vi "Central_Controller_KAFB.vi"() -> ()   [LabVIEW 2019]
uses:
  <vilib>/Modbus/master/Modbus Master.lvclass
  <vilib>/Modbus/master/Create Master Instance (TCP).vi
panel:
  in  "DER List":string[](array[string])=["Capstone", "Aquion", "Tesla", "Load Bank", "Motor 1", "Simpliphi 1", "LG Chem", "Outback 1", "Outback 2", "Sunny Island", "ESS", "Fuel Cells", "Sparkplug", "Fronius", "Suny Boy", "Motor 2"]
  out "data":T1
  in  "File Name":string
  out "error out 3":errorcluster
  in  "Folder":path=path "C:/Users/administrator.STONEEDGEPOWER/Desktop/Data"
  out "ALL Status":u16[](array[numeric])
  out "ALL AC RMS Line-Neutral Voltages":sgl[][](array[numeric])
  out "SYS Current Time":dbl format="%.3f"
  out "SYS DER Index":i32
  out "ALL Frequency":sgl[](array[numeric])
  out "ALL Control Method":string[](array[string])
  out "ALL Logged":bool[](array[boolean])
  out "ALL Through Variable":sgl[](array[numeric])
  out "ALL Across Variable":sgl[](array[numeric])
  out "ALL State of Charge":sgl[](array[numeric])
  out "ALL Reactive Power":sgl[](array[numeric])
  out "ALL Real Power":sgl[](array[numeric])
  out "ALL AC RMS Line-Line Average Voltage":sgl[][](array[numeric])
  in  "Tab Control Main":enum32{"Control", "Comms Control"}(tab)
  out "DER12 Flow":i32(ring)
  out "DER12State of Charge Figure":sgl(slide) scale=0.0..100.0
  out "DER12 State of Charge":sgl format="%#.1f"
  out "DER12 Real Power":sgl format="%.1f"
  in  "DER12 Login Button":bool
  out "DER12 Logged":bool
  out "DER12 DC Voltage":sgl format="%#.1f"
  out "DER12 AC Line-Line Voltage":sgl=209.57935 format="%.1f"
  out "DER12 State":string
  in  "DER12 Control Window Button":bool
  in  "DER12 Detail Window Button":bool
  out "DER11 State of Charge":sgl format="%#.1f"
  out "DER11 Flow":i32(ring)
  in  "DER11 Detail Window Button":bool
  out "DER11 State of Charge Figure":sgl(slide) scale=0.0..100.0
  in  "DER11 Login Button":bool
  out "DER11 Across Variable":sgl format="%#.2f"
  out "DER11 logged":bool
  out "DER11 AC Line-Line Votlage":sgl format="%.1f"
  out "DER11 Real Power":sgl format="%.1f"
  out "DER11 State":string
  in  "DER11 Control Window Button":bool
  out "DER10 Flow":i32(ring)
  out "DER10 State of Charge Figure":sgl(slide) scale=0.0..100.0
  out "DER10 State of Charge":sgl format="%#.1f"
  out "DER10 Real Power":sgl format="%.1f"
  in  "DER10 Login Button":bool
  out "DER10 Logged":bool
  out "DER10 DC Voltage":sgl format="%#.1f"
  out "DER10 AC Line-Line Voltage":sgl=209.57935 format="%.1f"
  out "DER10 State":string
  in  "DER10 Control Window Button":bool
  in  "DER10 Detail Window Button":bool
  out "DER9 State of Charge":sgl format="%#.1f"
  out "DER9 Flow":i32(ring)
  in  "DER9 Detail Window Button":bool
  out "DER9 State of Charge Figure":sgl(slide) scale=0.0..100.0
  in  "DER9 Login Button":bool
  out "DER9 Across Variable":sgl format="%#.2f"
  out "DER9 logged":bool
  out "DER9 AC Line-Line Votlage":sgl format="%.1f"
  out "DER9 Real Power":sgl format="%.1f"
  out "DER9 State":string
  in  "DER9 Control Window Button":bool
  out "DER8 Flow":i32(ring)
  out "DER8 State of Charge Figure":sgl(slide) scale=0.0..100.0
  out "DER8 State of Charge":sgl format="%#.1f"
  out "DER8 Real Power":sgl format="%.1f"
  in  "DER8 Login Button":bool
  out "DER8 Logged":bool
  out "DER8 DC Voltage":sgl format="%#.1f"
  out "DER8 AC Line-Line Voltage":sgl=209.57935 format="%.1f"
  out "DER8 State":string
  in  "DER8 Control Window Button":bool
  in  "DER8 Detail Window Button":bool
  out "DER7 State of Charge":sgl format="%#.1f"
  out "DER5 State of Charge":sgl format="%#.1f"
  out "DER7 Flow":i32(ring)
  in  "DER7 Detail Window Button":bool
  out "DER7 State of Charge Figure":sgl(slide) scale=0.0..100.0
  in  "DER7 Login Button":bool
  out "DER7 Across Variable":sgl format="%#.2f"
  out "DER7 logged":bool
  out "DER7 AC Line-Line Votlage":sgl format="%.1f"
  out "DER7 Real Power":sgl format="%.1f"
  out "DER7 State":string
  in  "DER7 Control Window Button":bool
  out "DER6 Flow":i32(ring)
  out "DER6 State of Charge Figure":sgl(slide) scale=0.0..100.0
  out "DER6 State of Charge":sgl format="%#.1f"
  out "DER6 Real Power":sgl format="%.1f"
  in  "DER6 Login Button":bool
  out "DER6 Logged":bool
  out "DER6 DC Voltage":sgl format="%#.1f"
  out "DER6 AC Line-Line Voltage":sgl=209.57935 format="%.1f"
  out "DER6 State":string
  in  "DER6 Control Window Button":bool
  in  "DER6 Detail Window Button":bool
  out "DER0 State of Charge":sgl format="%.1f"
  out "DER0 State of Charge Figure":sgl(slide) scale=0.0..100.0
  out "DER5 Flow":i32(ring)
  out "DER4 Flow":i32(ring)
  out "DER3 Flow":i32(ring)
  out "DER1 Flow":i32(ring)
  out "DER0 Flow":i32(ring)
  in  "DER2 Detail Window Button":bool
  in  "DER5 Detail Window Button":bool
  out "DER4 State of Charge Figure":sgl(slide) scale=0.0..100.0
  out "DER4 State of Charge":sgl format="%#.1f"
  out "DER4 Real Power":sgl format="%.1f"
  in  "DER15 Login Button":bool
  out "DER4 Logged":bool
  out "DER4 DC Voltage":sgl format="%#.1f"
  out "DER4 AC Line-Line Voltage":sgl=209.57935 format="%.1f"
  out "DER4 State":string
  out "DER5 State of Charge Figure":sgl(slide) scale=0.0..100.0
  in  "DER0 Login Button":bool
  in  "DER2 Login Button":bool
  in  "DER1 Login Button":bool
  out "DER1 State of Charge Figure":sgl(slide) scale=0.0..100.0
  out "DER1 Real Power":sgl format="%.1f"
  out "DER1 Reactive Power":sgl format="%#.1f"
  out "DER1 AC Line-Line Voltage":sgl format="%.1f"
  out "DER0 Real Power":sgl format="%#.1f"
  out "DER0 AC Line-Line Voltage":sgl format="%#.1f"
  out "DER2 AC Line-Line Voltage":sgl format="%.1f"
  out "DER2 Real Power":sgl format="%.1f"
  out "DER0 Logged":bool
  out "DER1 Logged":bool
  out "DER2 Logged":bool
  out "DER1 State of Charge":sgl format="%.1f"
  in  "DER3 Login Button":bool
  out "DER3 Logged":bool
  out "DER3 Real Power":sgl format="%#.1f"
  out "DER3 AC Line-Line Votlage":sgl format="%#.1f"
  in  "DER5 Login Button":bool
  out "DER5 Across Variable":sgl format="%#.2f"
  out "DER5 logged":bool
  out "DER5 AC Line-Line Votlage":sgl format="%.1f"
  out "DER5 Real Power":sgl format="%.1f"
  out "DER0 State":string
  out "DER1 State":string
  out "DER2 State":string
  out "DER3 State":string
  out "DER5 State":string
  in  "DER0 Control Window Button":bool
  in  "DER0 Detail Window Button":bool
  in  "DER1 Detail Window Button":bool
  in  "DER1 Control Window Button":bool
  in  "DER2 Control Window Button":bool
  in  "DER3 Control Window Button":bool
  in  "DER5 Control Window Button":bool
  in  "DER4 Control Window Button":bool
  in  "DER3 Detail Window Button":bool
  in  "DER4 Detail Window Button":bool
  out "DER2 Control Mode":string="Slave Mode Droops"
  out "DER1 Control Mode":string="Slave Mode Droops"
  out "DER2 Flow":i32(ring)
  out "DER0 Control Mode":string="Slave Mode Droops"
  in  "Tab Control Communications":enum32{"Page 1"}(tab)
  out "ALL Error Indicator":bool[](array[boolean])
  out "ALL DER Current Error":errorcluster[](array[cluster])
  out "ALL DER Final Error":errorcluster[](array[cluster])
  in  "IP Address List":string[](array[string])=["10.1.32.65", "10.1.32.32", "10.0.1.180", "10.0.1.202", "10.0.1.189", "10.0.1.188", "10.0.1.190", "10.0.1.187", "10.0.1.195", "10.0.1.191", "10.0.1.185", "10.0.1.181", "10.0.1.201", "10.0.1.192", "10.0.1.207", "10.0.1.196"]
  in  "DER Label Name":string[](array[string])=["DER0", "DER1", "DER2", "DER3", "DER4", "DER5", "DER6", "DER7", "DER8", "DER9", "DER10", "DER11", "DER12", "DER13", "DER14", "DER15"]
  out "SYS Iteration":i32
  in  "stop":bool
  out "SYS Status":string="Reading"
  out "SYS Case":i32
  in  "Read Array":bool[](array[boolean])
  # "DER0: Heila XX, Sinamics, 10.0.8.XX\nDER1: Heila XX, Socomec, 10.0.8.XX\nDER2: Heila XX, Alencon, 10.0.8.XX\nDER3: Heila XX, Polar Power, 10.0.8.XX\nDER4: Heila XX, Nanogrid 1 \nDER5: Heila XX, Nanogrid 2\nDER6: Heila XX, Nanogrid 3\nDER7: Heila XX, Nanogrid 4 \nDER8: Heila XX, Nanogrid 5\nDER9: Heila XX, Nanogrid 6\nDER10: Heila XX, Nanogrid 7 \nDER11: Heila XX, Nanogrid 8\nDER12: Heila XX, Nanogrid 9"
  # "Nanogrid"
  # "Generators"
  # "Battery"
  # "Nanogrid"
  # "Nanogrid"
  # "Nanogrid"
  # "Nanogrid"
  # "Schaefer"
  # "EPIC + Polar Power"
  # "Sinamics + Energport"
  # "Schaefer"
  # "Schaefer"
  # "Schaefer"
  # "Schaefer"
  # "Status:"
  # "Status:"
  # "Status:"
  # "Status:"
  # "Status:"
  # "Status:"
  # "Status:"
  # "Mode:"
  # "V"
  # "V"
  # "V"
  # "V"
  # "V"
  # "KAFB Microgrid in Real Time"
  # "SoC"
  # "%"
  # "SoC"
  # "%"
  # "SoC"
  # "%"
  # "SoC"
  # "%"
  # "SoC"
  # "%"
  # "SoC"
  # "%"
  # "kW"
  # "kW"
  # "kW"
  # "kW"
  # "kW"
  # "kW"
  # "kW"
  # "Inverter"
  # "Utility Grid"
  # "kW"
  # "V"
  # "V"
  # "V"
  # "V"
  # "V"
  # "V"
  # "V"
  # "Socomec"
  # "kVAr"
  # "V"
  # "Status:"
  # "Mode:"
  # "V ="
  # "V"
  # "f ="
  # "Hz"
  # "P ="
  # "W"
  # "Q ="
  # "VAr"
  # "kW"
  # "kW"
  # "kW"
  # "kW"
  # "kW"
  # "SoC"
  # "%"
  # "V"
  # "V"
  # "V"
  # "V"
  # "V"
  # "Nanogrid"
  # "Nanogrid"
  # "Nanogrid"
  # "Nanogrid"
  # "Solar"
  # "Sinexcel"
  # "Sinexcel"
  # "Sinexcel"
  # "Sinexcel"
  # "PV + Alencon"
  # "Status:"
  # "Status:"
  # "Status:"
  # "Status:"
  # "Status:"
  # "Mode:"
  # "V"
  # "V"
  # "V"
  # "V"
  # "SoC"
  # "%"
  # "SoC"
  # "%"
  # "SoC"
  # "%"
  # "SoC"
  # "%"
  # "Program"
  # "Controllable DERs"
  # "DER0: Heila XX, Sinamics, 10.1.32.65\nDER1: Heila XX, Socomec, 10.1.32.32\nDER2: Heila XX, Alencon, 10.1.32.XX\nDER3: Heila XX, Polar Power, 10.1.32.XX\nDER4: Heila XX, Nanogrid 1, 10.1.32.45 \nDER5: Heila XX, Nanogrid 2, 10.1.32.67\nDER6: Heila XX, Nanogrid 3, 10.1.32.70\nDER7: Heila XX, Nanogrid 4, 10.1.32.100\nDER8: Heila XX, Nanogrid 5, 10.1.32.68\nDER9: Heila XX, Nanogrid 6, 10.1.32.38\nDER10: Heila XX, Nanogrid 7, 10.1.32.43\nDER11: Heila XX, Nanogrid 8\nDER12: Heila XX, Nanogrid 9"
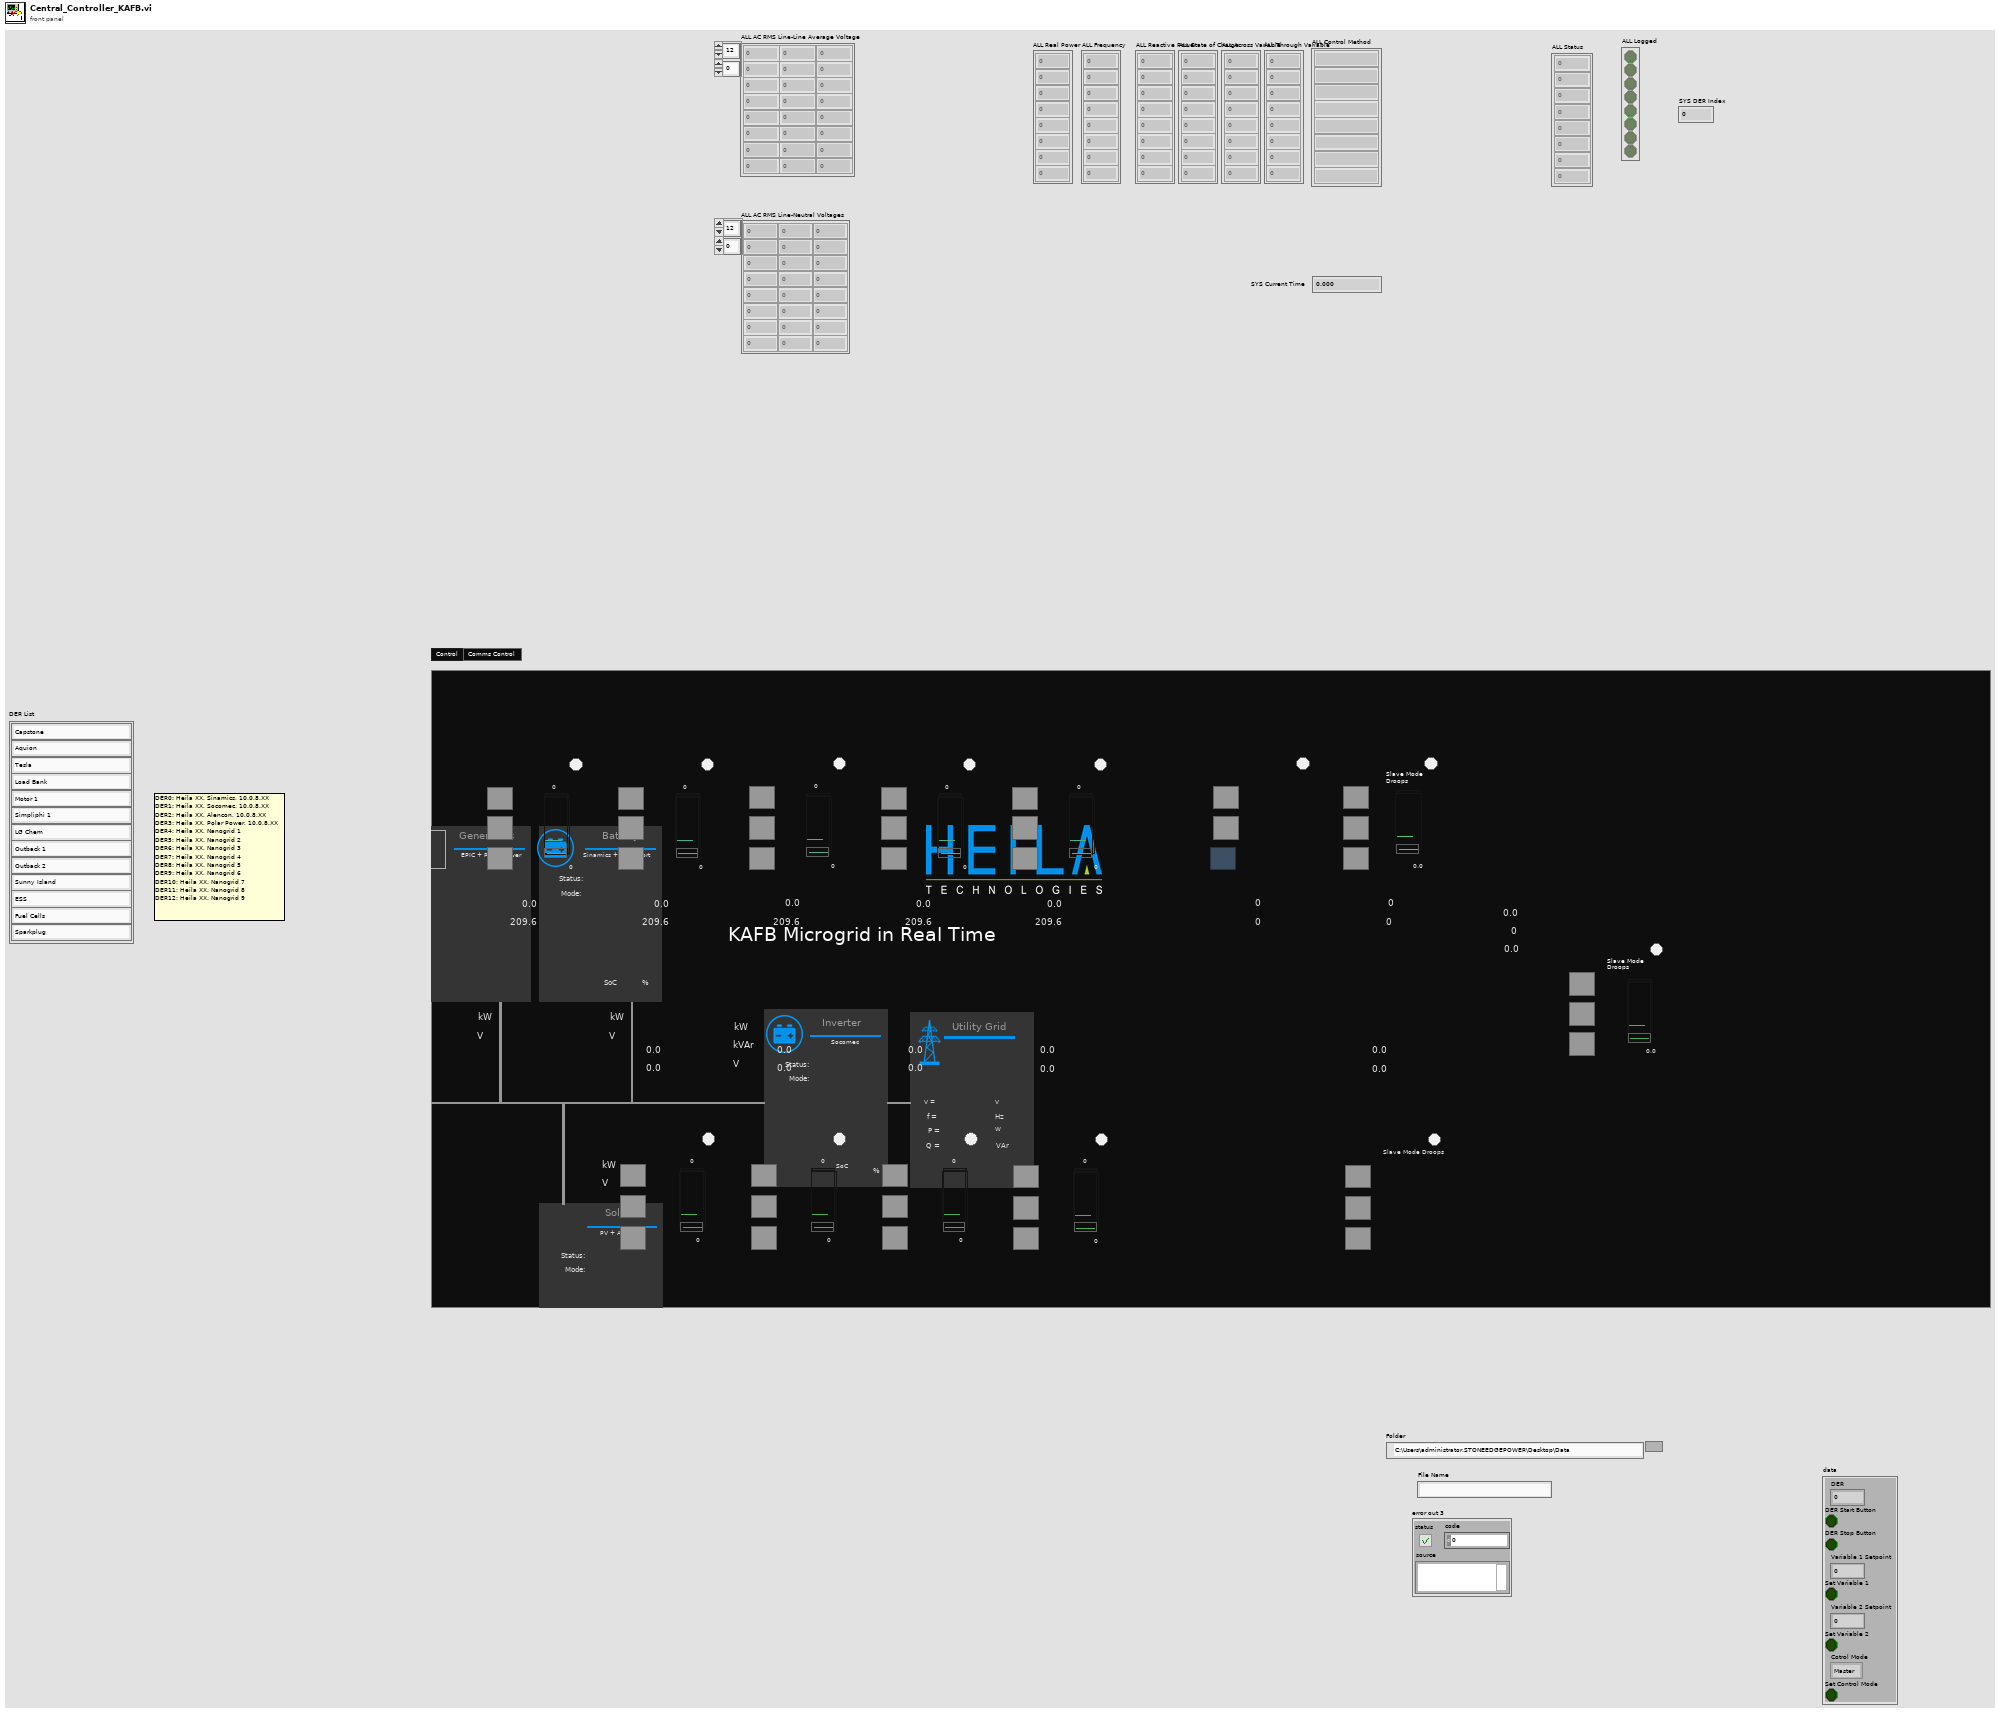
[diagram p1: front panel]
types:
  T1 = cluster{"DER":i32, "DER Start Button":bool, "DER Stop Button":bool, "Variable 1 Setpoint":sgl, "Set Variable 1":bool, "Variable 2 Setpoint":sgl, "Set Variable 2":bool, "Cotrol Mode":enum16{"Master", "Slave"}, "Set Control Mode":bool}
  T2 = enum16{"open", "replace", "create", "open or create", "replace or create", "replace or create with confirmation"}
  T3 = cluster{"Modbus master out":refnum<class "Modbus Master.lvclass">, "error out":errorcluster}[]
  T4 = enum32{"Invalid", "Standard", "Closed", "Hidden", "Minimized", "Maximized"}
  T5 = cluster{"Modbus master out":refnum<class "Modbus Master.lvclass">, "error out":errorcluster}
  T6 = enum32{"Bad", "Idle", "Run top level", "Running"}
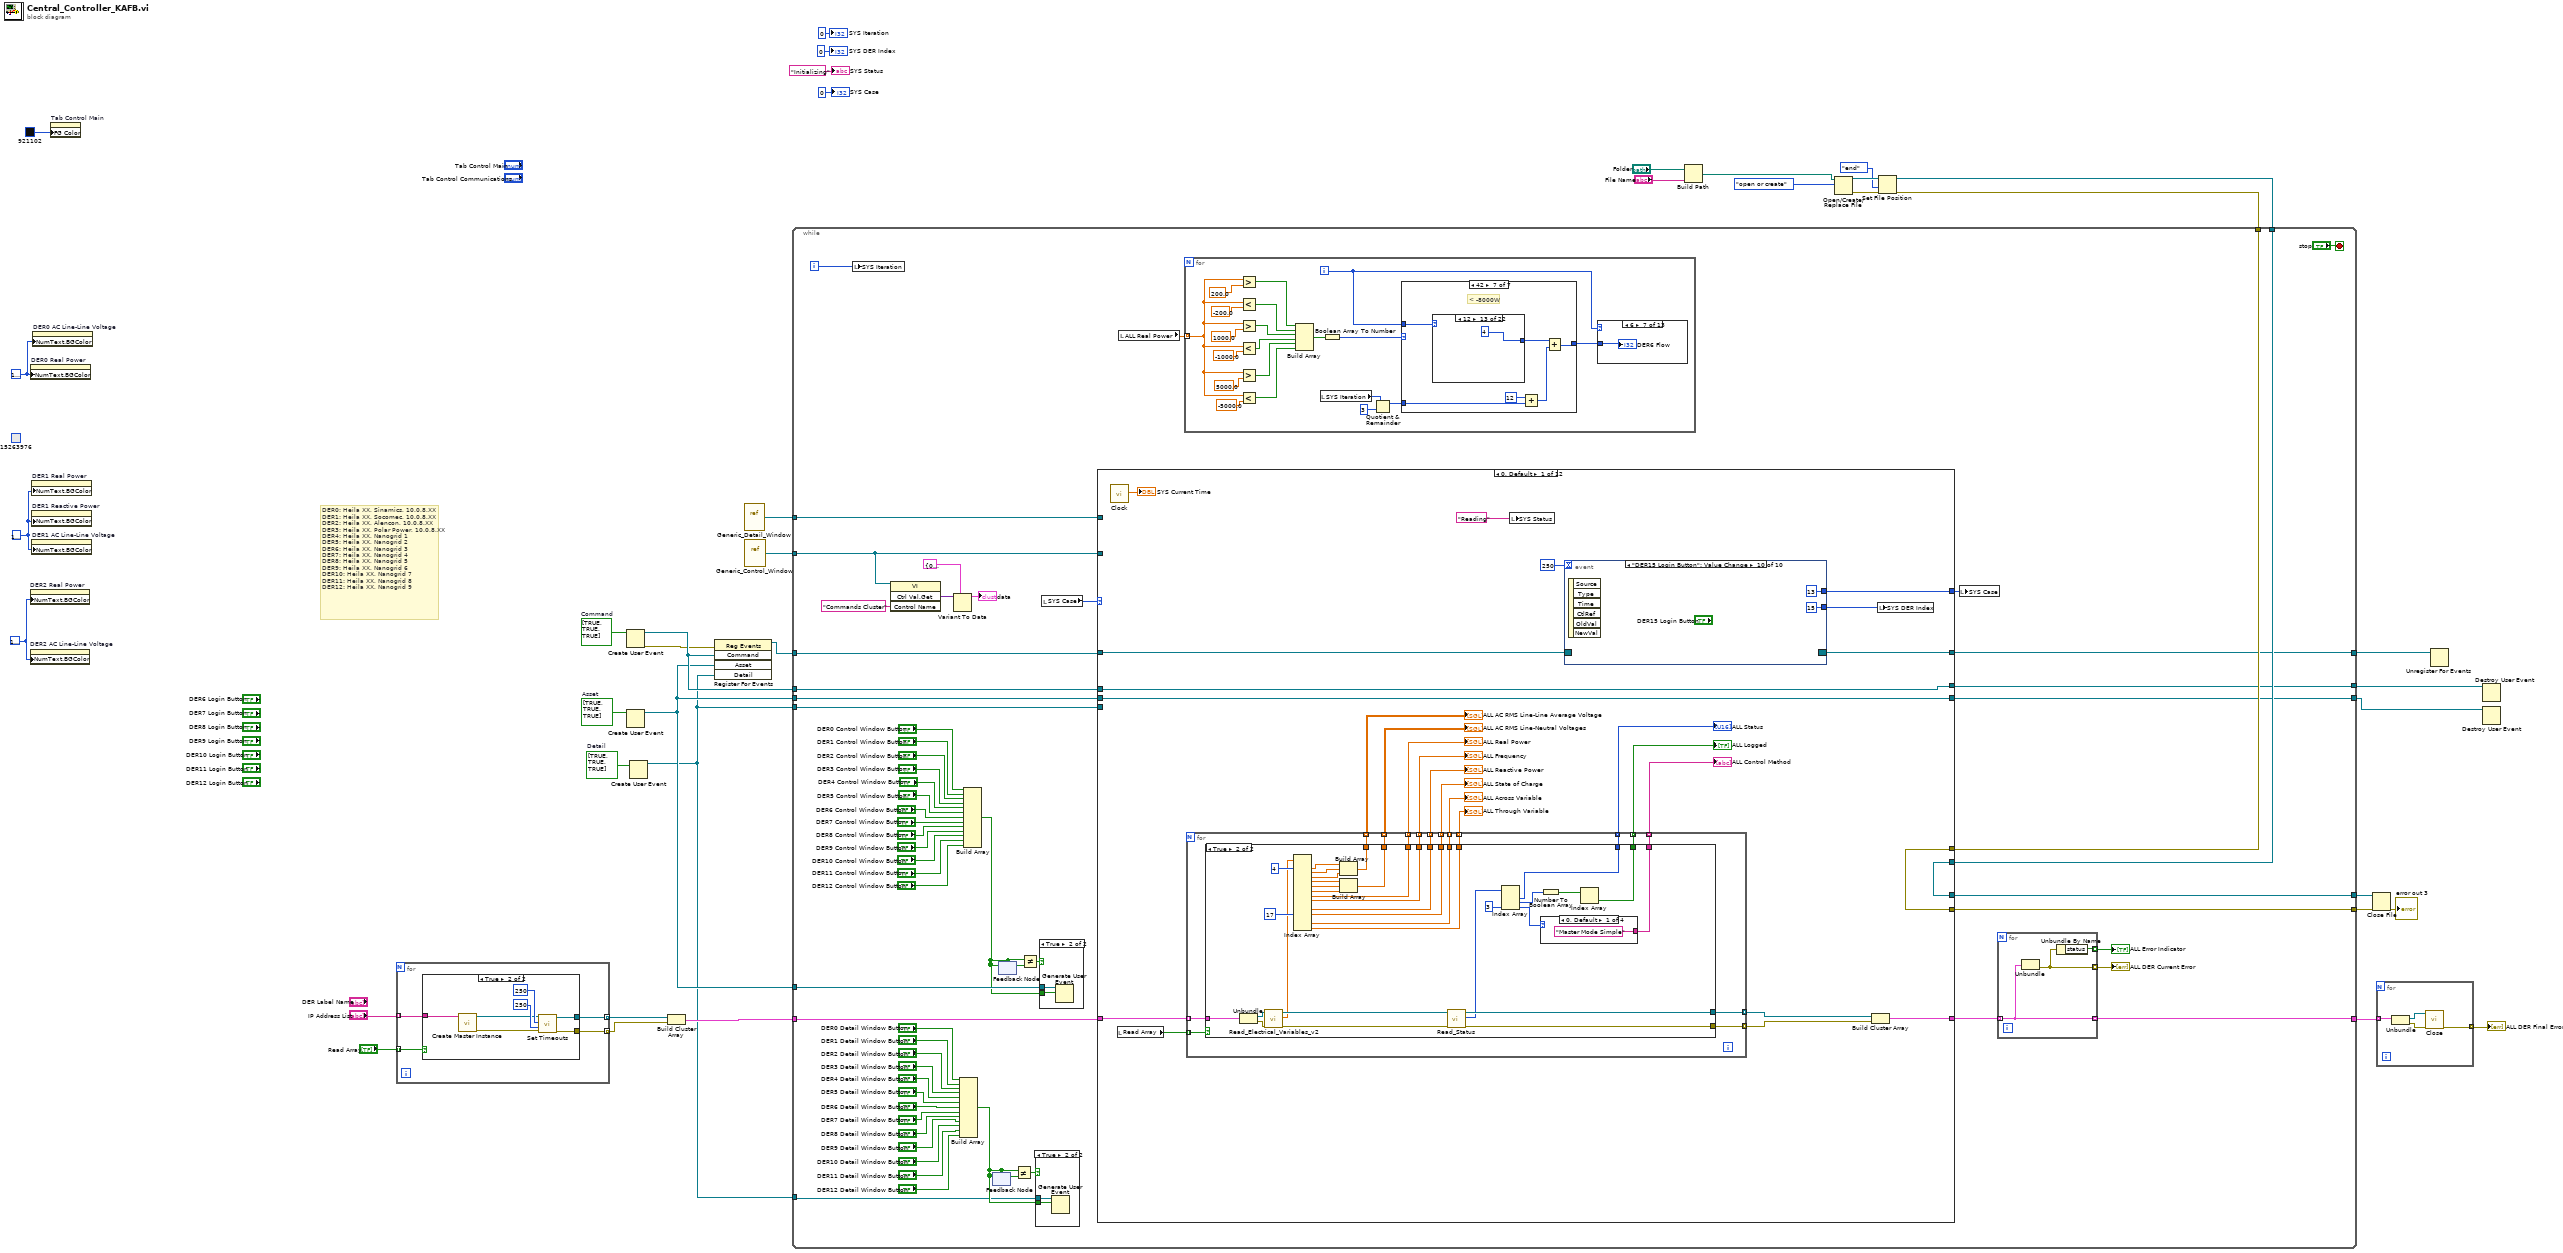
[diagram p0: block diagram]
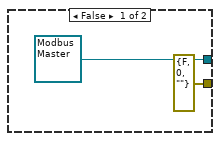
[diagram p2: hidden frame]
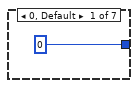
[diagram p5: hidden frame]
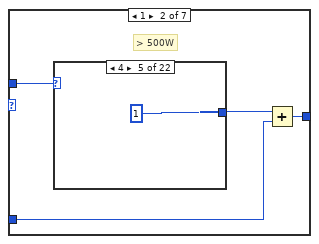
[diagram p6: hidden frame]
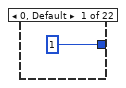
[diagram p7: hidden frame]
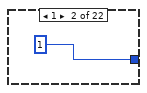
[diagram p8: hidden frame]
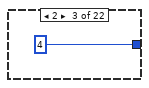
[diagram p9: hidden frame]
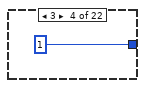
[diagram p10: hidden frame]
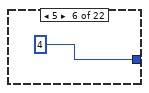
[diagram p11: hidden frame]
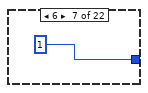
[diagram p12: hidden frame]
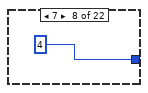
[diagram p13: hidden frame]
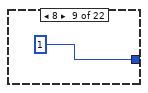
[diagram p14: hidden frame]
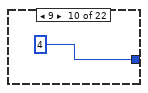
[diagram p15: hidden frame]
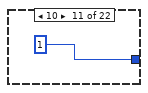
[diagram p16: hidden frame]
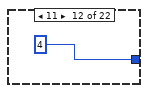
[diagram p17: hidden frame]
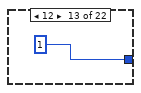
[diagram p18: hidden frame]
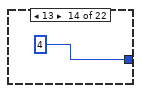
[diagram p19: hidden frame]
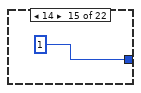
[diagram p20: hidden frame]
diagram:
  w4 = bool[] [TRUE, TRUE, TRUE]  # Detail
  w10 = bool[] [TRUE, TRUE, TRUE]  # Asset
  w13 = bool[] [TRUE, TRUE, TRUE]  # Command
  w36 = u32 16777216
  w37 = u32 16777216
  w38 = u32 16777216
  (unwired) u32 15263976
  # "DER0: Heila XX, Sinamics, 10.0.8.XX\nDER1: Heila XX, Socomec, 10.0.8.XX\nDER2: Heila XX, Alencon, 10.0.8.XX\nDER3: Heila XX, Polar Power, 10.0.8.XX\nDER4: Heila XX, Nanogrid 1 \nDER5: Heila XX, Nanogrid 2\nDER6: Heila XX, Nanogrid 3\nDER7: Heila XX, Nanogrid 4 \nDER8: Heila XX, Nanogrid 5\nDER9: Heila XX, Nanogrid 6\nDER10: Heila XX, Nanogrid 7 \nDER11: Heila XX, Nanogrid 8\nDER12: Heila XX, Nanogrid 9"
  n1 = property on="DER2 Real Power" class="DigNum (strict)"("NumText.BGColor"=w36) -> ()  [unwired: 2 in, 2 out]
  n2 = property on="DER2 AC Line-Line Voltage" class="DigNum (strict)"("NumText.BGColor"=w36) -> ()  [unwired: 2 in, 2 out]
  n3 = property on="DER0 Real Power" class="DigNum (strict)"("NumText.BGColor"=w38) -> ()  [unwired: 2 in, 2 out]
  n4 = property on="DER1 Real Power" class="DigNum (strict)"("NumText.BGColor"=w37) -> ()  [unwired: 2 in, 2 out]
  n5 = property on="DER1 Reactive Power" class="DigNum (strict)"("NumText.BGColor"=w37) -> ()  [unwired: 2 in, 2 out]
  n6 = property on="DER1 AC Line-Line Voltage" class="DigNum (strict)"("NumText.BGColor"=w37) -> ()  [unwired: 2 in, 2 out]
  n7 = property on="DER0 AC Line-Line Voltage" class="DigNum (strict)"("NumText.BGColor"=w38) -> ()  [unwired: 2 in, 2 out]
  n8 = property on="Tab Control Main" class="TabCtl (strict)"("FG Color"=u32 921102) -> ()  [unwired: 2 in, 2 out]
  n9 = for {
    tunnel: "IP Address List" -> [w44] mode=indexing
    tunnel: [w43] -> w35 mode=indexing
    tunnel: [w42] -> w34 mode=indexing
    tunnel: "Read Array" -> [w41] mode=indexing
    n10 = case shown="True" w41 {
      tunnel: w44 -> [_ w53]
      tunnel: [refnum<class "Modbus Master.lvclass"> refnum ("Modbus master out") w50] -> w43
      tunnel: [errorcluster {"status"=FALSE, "code"=0, "source"=""} ("error out") w49] -> w42
      frame False {
      }
      frame True {
        n11 = call-poly <vilib>:"Create Master Instance.vi"("address"=w53) -> ("error out"=w47:errorcluster, "TCP master instance"=w48:refnum<class "Modbus Master.lvclass">)  [unwired: 9 in]
        n12 = call <vilib>:"Set Timeouts.vi"("error in (no error)"=w47, "write operation timeout (ms)"=250 ("Write Timeout"), "read operation timeout (ms)"=250 ("Read Timeout"), "Modbus master in"=w48) -> ("error out"=w49:errorcluster, "Modbus master out"=w50:refnum<class "Modbus Master.lvclass">)  [unwired: 6 in]
      }
    }
  }
  n13 = Create User Event(user event datatype=w13) -> (user event=w11:refnum<user-event>, error out=w7:errorcluster)  [unwired: 1 in]
  n14 = Create User Event(user event datatype=w10) -> (user event=w6:refnum<user-event>)  [unwired: 1 in, 1 out]
  n15 = Create User Event(user event datatype=w4) -> (user event=w2:refnum<user-event>)  [unwired: 1 in, 1 out]
  n16 = Build Cluster Array(w35, w34) -> (w33:T3)
  n17 = register-events(error in=w7, w11, w6, w2) -> (reference out=w12:refnum<event-registration>)  [unwired: 1 in, 1 out]
  n18 = vi-ref "Generic_Detail_Window.vi"() -> (w3:refnum<vi>)
  n19 = vi-ref "Generic_Control_Window.vi"() -> (w14:refnum<vi>)
  n20 = Build Path(base path="Folder", name or relative path="File Name") -> (appended path=w15:path)
  n21 = Open/Create/Replace File(file path (use dialog)=w15, operation (0:open)=T2."open or create") -> (refnum out=w25:refnum<file>, error out=w24:errorcluster)  [unwired: 4 in, 1 out]
  n22 = Set File Position(refnum=w25, from (0:start)=enum16{"start", "end", "current"}."end", error in=w24) -> (refnum out=w19:refnum<file>, error out=w18:errorcluster)  [unwired: 1 in]
  n23 = while {
    tunnel: w33 -> [w112]
    tunnel: [w108] -> w27
    tunnel: [w106] -> w22
    tunnel: [w105] -> w21
    tunnel: w19 -> [w104]
    tunnel: w18 -> [w103]
    tunnel: w14 -> [w83]
    tunnel: w11 -> [w101]
    tunnel: w6 -> [w92]
    tunnel: [w89] -> w8
    tunnel: w6 -> [w88]
    tunnel: [w87] -> w5
    tunnel: w12 -> [w102]
    tunnel: [w90] -> w9
    tunnel: w2 -> [w73]
    tunnel: w3 -> [w72]
    tunnel: w2 -> [w71]
    i -> [w54]
    stop <- "stop" stop-if-true
    n24 = local write "SYS Iteration"(w54) -> ()
    n25 = invoke class="VI" method="Ctrl Val.Get"(reference=w83, "Control Name"="Commands Cluster") -> ("Get Control Value Variant"=w100:variant)  [unwired: 2 in, 3 out]
    n26 = Variant To Data(type=T1 {"DER"=0, "DER Start Button"=FALSE, "DER Stop Button"=FALSE, "Variable 1 Setpoint"=0.0, "Set Variable 1"=FALSE, "Variable 2 Setpoint"=0.0, "Set Variable 2"=FALSE, "Cotrol Mode"=enum."Slave", "Set Control Mode"=FALSE} ("Commands Cluster 2"), Variant=w100) -> (data=→"data":T1)  [unwired: 1 in, 1 out]
    n27 = Build Array("DER0 Detail Window Button", "DER1 Detail Window Button", "DER2 Detail Window Button", "DER3 Detail Window Button", "DER4 Detail Window Button", "DER5 Detail Window Button", "DER6 Detail Window Button", "DER7 Detail Window Button", "DER8 Detail Window Button", "DER9 Detail Window Button", "DER10 Detail Window Button", "DER11 Detail Window Button", "DER12 Detail Window Button") -> (w75:bool[])
    n28 = Build Array("DER0 Control Window Button", "DER1 Control Window Button", "DER2 Control Window Button", "DER3 Control Window Button", "DER4 Control Window Button", "DER5 Control Window Button", "DER6 Control Window Button", "DER7 Control Window Button", "DER8 Control Window Button", "DER9 Control Window Button", "DER10 Control Window Button", "DER11 Control Window Button", "DER12 Control Window Button") -> (w91:bool[])
    n29 = feedback #1(w75) -> (w76:bool[])
    n30 = feedback-in #1(w75) -> ()
    n31 = feedback-in #2(w91) -> ()
    n32 = feedback #2(w91) -> (w93:bool[])
    n33 = Not Equal?(x=w75, y=w76) -> (x != y?=w74:bool)
    n34 = Not Equal?(x=w91, y=w93) -> (x != y?=w86:bool)
    n35 = case shown="True" w74 {
      tunnel: w73 -> [_ w116]
      tunnel: w75 -> [_ w115]
      frame False {
      }
      frame True {
        n36 = Generate User Event(user event=w116, event data cluster=w115) -> ()  [unwired: 2 in, 2 out]
      }
    }
    n37 = case shown="True" w86 {
      tunnel: w92 -> [_ w118]
      tunnel: w91 -> [_ w117]
      frame False {
      }
      frame True {
        n38 = Generate User Event(user event=w118, event data cluster=w117) -> ()  [unwired: 2 in, 2 out]
      }
    }
    n39 = local read "SYS Case"() -> (w113:i32)
    n40 = case shown="0, Default" w113 {
      tunnel: [w345 2 0 0 0 0 0 0 0 0 w770 w800] -> w82
      tunnel: [w340 w467 w635 w640 w654 w671 w704 w717 w735 w754 w774 w802] -> w111
      tunnel: w112 -> [w343 w467 w635 w642 w655 w675 w705 w716 w736 w755 w774 w802]
      tunnel: [w326 _ w632 _ _ _ _ _ _ _ _ _] -> w106
      tunnel: [w327 _ w631 _ _ _ _ _ _ _ _ _] -> w105
      tunnel: w104 -> [w326 _ w630 _ _ _ _ _ _ _ _ _]
      tunnel: w103 -> [w327 _ w629 _ _ _ _ _ _ _ _ _]
      tunnel: w83 -> [_ _ _ _ _ _ _ _ _ _ w771 _]
      tunnel: w102 -> [w325 w455 w625 _ _ _ _ _ _ _ _ _]
      tunnel: [w324 w455 w625 _ _ _ _ _ _ _ _ _] -> w90
      tunnel: w101 -> [w323 _ _ _ _ _ _ _ _ _ w773 _]
      tunnel: [w323 _ _ _ _ _ _ _ _ _ _ _] -> w89
      tunnel: w88 -> [w322 _ _ _ _ _ _ _ _ _ _ _]
      tunnel: [w322 _ _ _ _ _ _ _ _ _ _ _] -> w87
      tunnel: w72 -> [_ _ _ _ _ _ _ _ _ _ _ w799]
      tunnel: w71 -> [_ _ _ _ _ _ _ _ _ _ _ _]
      frame 0, Default {
        n41 = call "Clock.vi"() -> ("SYS Current Time"=→"SYS Current Time":dbl)  [unwired: 11 in]
        n42 = local read "Read Array"() -> (w320:bool[])
        n43 = for {
          tunnel: w343 -> [w361] mode=indexing
          tunnel: [w360] -> w342 mode=indexing
          tunnel: [w359] -> w341 mode=indexing
          tunnel: [w349] -> w338 mode=indexing
          tunnel: [w358] -> w337 mode=indexing
          tunnel: [w348] -> w339 mode=indexing
          tunnel: [w357] -> w336 mode=indexing
          tunnel: [w353] -> w335 mode=indexing
          tunnel: [w352] -> w334 mode=indexing
          tunnel: [w356] -> w332 mode=indexing
          tunnel: [w355] -> w333 mode=indexing
          tunnel: [w354] -> w331 mode=indexing
          tunnel: [w351] -> w329 mode=indexing
          tunnel: [w350] -> w328 mode=indexing
          tunnel: w320 -> [w347] mode=indexing
          n44 = case shown="True" w347 {
            tunnel: w361 -> [w364 w401]
            tunnel: [w363 w396] -> w360
            tunnel: [w362 w395] -> w359
            tunnel: [w367 w387] -> w358
            tunnel: [w367 w386] -> w357
            tunnel: ["N/A" w385] -> w356
            tunnel: [FALSE w383] -> w355
            tunnel: [w367 w382] -> w354
            tunnel: [w367 w381] -> w353
            tunnel: [w367 w380] -> w352
            tunnel: [w368 w376] -> w351
            tunnel: [u16 1 ("register") w375] -> w350
            tunnel: [w367 w374] -> w349
            tunnel: [w368 w370] -> w348
            frame False {
              w367 = sgl 0.0
              w368 = sgl[] [0.0, 0.0, 0.0]
              n45 = Unbundle(w364) -> ("Modbus master out"=w363:refnum<class "Modbus Master.lvclass">, "error out"=w362:errorcluster)
            }
            frame True {
              n46 = Unbundle(w401) -> ("Modbus master out"=w400:refnum<class "Modbus Master.lvclass">, "error out"=w399:errorcluster)
              n47 = call "Read_Electrical_Variables_v2.vi"("error in (no error)"=w399, "Modbus master in"=w400) -> ("error out"=w397:errorcluster, "Variables"=w392:sgl[], "Modbus master out"=w398:refnum<class "Modbus Master.lvclass">)  [unwired: 7 in]
              n48 = Index Array(array=w392, index #1=4, index #11=17 ("index")) -> (element #1=w373:sgl, element #2=w372:sgl, element #3=w371:sgl, element #4=w379:sgl, element #5=w378:sgl, element #6=w377:sgl, element #7=w374:sgl, element #8=w382:sgl, element #10=w387:sgl, element #11=w386:sgl, element #13=w381:sgl, element #14=w380:sgl)  [unwired: 12 in, 2 out]
              n49 = Build Array(w373, w372, w371) -> (w370:sgl[])
              n50 = Build Array(w379, w378, w377) -> (w376:sgl[])
              n51 = call "Read_Status.vi"("error in (no error)"=w397, "Modbus master in"=w398) -> ("error out"=w395:errorcluster, "Variables"=w390:u16[], "Modbus master out"=w396:refnum<class "Modbus Master.lvclass">)  [unwired: 7 in]
              n52 = Index Array(array=w390, index #3=3) -> (element #1=w375:u16, element #2=w389:u16, element #3=w388:u16)  [unwired: 2 in]
              n53 = case shown="0, Default" w388 {
                tunnel: ["Master Mode Simple" "Slave Mode Simple" "Master Mode Droops" "Slave Mode Droops"] -> w385
                frame 0, Default {
                }
                frame 1 {
                }
                frame 2 {
                }
                frame 3 {
                }
              }
              n54 = Number To Boolean Array(number=w389) -> (Boolean array=w384:bool[])
              n55 = Index Array(array=w384) -> (element=w383:bool)  [unwired: 1 in]
            }
          }
        }
        "ALL AC RMS Line-Line Average Voltage" <- w339
        "ALL Real Power" <- w338
        "ALL Reactive Power" <- w337
        "ALL State of Charge" <- w336
        "ALL Across Variable" <- w335
        "ALL Through Variable" <- w334
        "ALL Logged" <- w333
        "ALL Control Method" <- w332
        "ALL Frequency" <- w331
        "ALL AC RMS Line-Neutral Voltages" <- w329
        "ALL Status" <- w328
        n56 = local write "SYS Status"("Reading") -> ()
        n57 = event shown="[9] \"DER15 Login Button\": Value Change" {
          selector: w325 -> [w406 _ _ _ w442 _ _ _ _ _]
          dyn-events: [w406 _ _ _ w442 _ _ _ _ _] -> w324
          timeout: 250 -> [_ _ _ _ _ _ _ _ _ _]
          tunnel: [1 w411 w422 w432 13 13 13 13 13 13] -> w345
          tunnel: [0 w410 w420 w431 0 1 2 3 5 15 ("DER")] -> w330
          event Timeout {
            n58 = event-data() -> ()  [unwired: 1 in, 1 out]
          }
          event User Event {
            n59 = event-data() -> ("Asset"=w415:bool[])  [unwired: 1 in]
            n60 = Search 1D Array(1D array=w415, element=TRUE) -> (index of element=w409:i32)  [unwired: 1 in]
            n61 = Equal?(x=w409, y=-1) -> (x = y?=w412:bool)
            n62 = case shown="False" w412 {
              tunnel: [1000 0] -> w411
              tunnel: [w416 0 ("index of element")] -> w410
              tunnel: w409 -> [w416 _]
              frame False {
              }
              frame True {
              }
            }
          }
          event User Event {
            n63 = event-data() -> ("Command"=w423:bool[])  [unwired: 1 in]
            n64 = Boolean Array To Number(Boolean array=w423) -> (number=w424:u32)
            n65 = case shown="0, Default" w424 {
              tunnel: [0 11 12 14 15 500] -> w422
              frame 0, Default {
              }
              frame 1 {
              }
              frame 2 {
              }
              frame 4 {
              }
              frame 8 {
              }
              frame 16 {
              }
            }
            n66 = local read "data"() -> (w421:T1)
            n67 = Unbundle By Name(w421) -> ("DER"=w420:i32)
          }
          event User Event {
            n68 = event-data() -> ("Detail"=w436:bool[])  [unwired: 1 in]
            n69 = Search 1D Array(1D array=w436, element=TRUE) -> (index of element=w433:i32)  [unwired: 1 in]
            n70 = Equal?(x=w433, y=-1) -> (x = y?=w434:bool)
            n71 = case shown="False" w434 {
              tunnel: [1001 0] -> w432
              tunnel: [w438 0 ("index of element")] -> w431
              tunnel: w433 -> [w438 _]
              frame False {
              }
              frame True {
              }
            }
          }
          event "DER0 Login Button": Value Change {
            n72 = event-data() -> ()  [unwired: 1 in, 1 out]
          }
          event "DER1 Login Button": Value Change {
            n73 = event-data() -> ()  [unwired: 1 in, 1 out]
          }
          event "DER2 Login Button": Value Change {
            n74 = event-data() -> ()  [unwired: 1 in, 1 out]
          }
          event "DER3 Login Button": Value Change {
            n75 = event-data() -> ()  [unwired: 1 in, 1 out]
          }
          event "DER5 Login Button": Value Change {
            n76 = event-data() -> ()  [unwired: 1 in, 1 out]
          }
          event "DER15 Login Button": Value Change {
            n77 = event-data() -> ()  [unwired: 1 in, 6 out]
          }
        }
        n78 = Build Cluster Array(w342, w341) -> (w340:T3)
        n79 = local write "SYS DER Index"(w330) -> ()
      }
      frame 1 {
        # "DER0: Heila XX, Sinamics, 10.0.8.XX\nDER1: Heila XX, Socomec, 10.0.8.XX\nDER2: Heila XX, Alencon, 10.0.8.XX\nDER3: Heila XX, Polar Power, 10.0.8.XX\nDER4: Heila XX, Nanogrid 1 \nDER5: Heila XX, Nanogrid 2\nDER6: Heila XX, Nanogrid 3\nDER7: Heila XX, Nanogrid 4 \nDER8: Heila XX, Nanogrid 5\nDER9: Heila XX, Nanogrid 6\nDER10: Heila XX, Nanogrid 7 \nDER11: Heila XX, Nanogrid 8\nDER12: Heila XX, Nanogrid 9"
        n80 = local read "ALL AC RMS Line-Line Average Voltage"() -> (w466:sgl[][])
        n81 = local read "ALL Real Power"() -> (w465:sgl[])
        n82 = local read "ALL Frequency"() -> (w459:sgl[])
        n83 = local read "ALL Reactive Power"() -> (w464:sgl[])
        n84 = local read "ALL State of Charge"() -> (w463:sgl[])
        n85 = local read "ALL Across Variable"() -> (w458:sgl[])
        n86 = local read "ALL Through Variable"() -> (w457:sgl[])
        n87 = local read "ALL Status"() -> (w462:u16[])
        n88 = local read "ALL Logged"() -> (w461:bool[])
        n89 = local read "ALL Control Method"() -> (w460:string[])
        n90 = local read "ALL AC RMS Line-Neutral Voltages"() -> (w456:sgl[][])
        n91 = for {
          tunnel: w466 -> [w482] mode=indexing
          tunnel: w465 -> [w481] mode=indexing
          tunnel: w464 -> [w480] mode=indexing
          tunnel: w463 -> [w479] mode=indexing
          tunnel: w462 -> [w472] mode=indexing
          tunnel: w461 -> [w478] mode=indexing
          tunnel: w460 -> [w477] mode=indexing
          tunnel: w459 -> [w476] mode=indexing
          tunnel: w458 -> [w475] mode=indexing
          tunnel: w457 -> [w474] mode=indexing
          tunnel: w456 -> [w473] mode=indexing
          i -> [w483]
          n92 = case shown="5" w472 {
            tunnel: ["Operating" "Off" "Sleeping" "Starting" "Stopping" "5: Busy" "6: N/A" "Fault" "Standby" "Generic Failure"] -> w471
            frame 0, Default {
            }
            frame 1 {
            }
            frame 2 {
            }
            frame 3 {
            }
            frame 4 {
            }
            frame 5 {
            }
            frame 6 {
            }
            frame 7 {
            }
            frame 8 {
            }
            frame 65535 {
            }
          }
          n93 = case shown="0, Default" w483 {
            tunnel: w482 -> [w498 w505 w520 w531 w539 w550 w561 w573 w583 w596 w606 _ _]
            tunnel: w481 -> [w503 w515 w524 w532 w544 w557 w564 w574 w584 w594 w607 _ _]
            tunnel: w480 -> [_ w511 _ _ _ _ _ _ _ _ _ _ _]
            tunnel: w479 -> [w496 w518 _ _ w542 w549 w570 w579 w589 w600 w611 w618 w619]
            tunnel: w478 -> [w504 w517 w527 w529 w547 w559 w567 w578 w592 w603 w613 w617 w620]
            tunnel: w477 -> [w494 w516 w528 _ _ _ _ _ _ _ _ w616 _]
            tunnel: w476 -> [_ _ _ _ _ _ _ _ _ _ _ _ _]
            tunnel: w475 -> [_ _ _ _ w546 w558 w569 w580 w590 w601 w614 w615 w622]
            tunnel: w474 -> [_ _ _ _ _ _ _ _ _ _ _ _ _]
            tunnel: w473 -> [_ _ _ _ _ _ _ _ _ _ _ _ _]
            tunnel: w471 -> [w495 w509 w519 w530 w548 w554 w568 w581 w591 w602 w612 _ w621]
            frame 0, Default {
              n94 = Add Array Elements(numeric array=w498) -> (sum=w501:sgl)
              n95 = Divide(x=w503, y=sgl 1000.0) -> (x/y=→"DER0 Real Power":sgl)
              n96 = Divide(x=w501, y=3.0) -> (x/y=→"DER0 AC Line-Line Voltage":dbl)
              "DER0 Logged" <- w504
              "DER0 State" <- w495
              "DER0 State of Charge Figure" <- w496
              "DER0 State of Charge" <- w496
              "DER0 Control Mode" <- w494
            }
            frame 1 {
              n97 = Add Array Elements(numeric array=w505) -> (sum=w508:sgl)
              n98 = Divide(x=w508, y=3.0) -> (x/y=→"DER1 AC Line-Line Voltage":dbl)
              n99 = Divide(x=w511, y=sgl 1000.0) -> (x/y=→"DER1 Reactive Power":sgl)
              n100 = Divide(x=w515, y=sgl 1000.0) -> (x/y=→"DER1 Real Power":sgl)
              "DER1 State of Charge" <- w518
              "DER1 State of Charge Figure" <- w518
              "DER1 Logged" <- w517
              "DER1 Control Mode" <- w516
              "DER1 State" <- w509
            }
            frame 2 {
              n101 = Add Array Elements(numeric array=w520) -> (sum=w523:sgl)
              n102 = Divide(x=w523, y=3.0) -> (x/y=→"DER2 AC Line-Line Voltage":dbl)
              n103 = Divide(x=w524, y=sgl 1000.0) -> (x/y=→"DER2 Real Power":sgl)
              "DER2 Logged" <- w527
              "DER2 Control Mode" <- w528
              "DER2 State" <- w519
            }
            frame 3 {
              n104 = Divide(x=w532, y=1000.0) -> (x/y=→"DER3 Real Power":dbl)
              n105 = Add Array Elements(numeric array=w531) -> (sum=w537:sgl)
              n106 = Divide(x=w537, y=3.0) -> (x/y=→"DER3 AC Line-Line Votlage":dbl)
              "DER3 Logged" <- w529
              "DER3 State" <- w530
            }
            frame 4 {
              n107 = Add Array Elements(numeric array=w539) -> (sum=w541:sgl)
              n108 = Divide(x=w544, y=sgl 1000.0) -> (x/y=→"DER4 Real Power":sgl)
              n109 = Divide(x=w541, y=3.0) -> (x/y=→"DER4 AC Line-Line Voltage":dbl)
              "DER4 DC Voltage" <- w546
              "DER4 State" <- w548
              "DER4 Logged" <- w547
              "DER4 State of Charge" <- w542
              "DER4 State of Charge Figure" <- w542
            }
            frame 5 {
              n110 = Divide(x=w557, y=sgl 1000.0) -> (x/y=→"DER5 Real Power":sgl)
              n111 = Add Array Elements(numeric array=w550) -> (sum=w553:sgl)
              n112 = Divide(x=w553, y=1.0) -> (x/y=→"DER5 AC Line-Line Votlage":dbl)
              "DER5 Across Variable" <- w558
              "DER5 logged" <- w559
              "DER5 State of Charge Figure" <- w549
              "DER5 State" <- w554
              "DER5 State of Charge" <- w549
            }
            frame 6 {
              n113 = Add Array Elements(numeric array=w561) -> (sum=w563:sgl)
              n114 = Divide(x=w564, y=sgl 1000.0) -> (x/y=→"DER6 Real Power":sgl)
              n115 = Divide(x=w563, y=1.0) -> (x/y=→"DER6 AC Line-Line Voltage":dbl)
              "DER6 State" <- w568
              "DER6 DC Voltage" <- w569
              "DER6 Logged" <- w567
              "DER6 State of Charge" <- w570
              "DER6 State of Charge Figure" <- w570
            }
            frame 7 {
              n116 = Add Array Elements(numeric array=w573) -> (sum=w576:sgl)
              n117 = Divide(x=w576, y=1.0) -> (x/y=→"DER7 AC Line-Line Votlage":dbl)
              n118 = Divide(x=w574, y=sgl 1000.0) -> (x/y=→"DER7 Real Power":sgl)
              "DER7 State of Charge Figure" <- w579
              "DER7 Across Variable" <- w580
              "DER7 State" <- w581
              "DER7 State of Charge" <- w579
              "DER7 logged" <- w578
            }
            frame 8 {
              n119 = Add Array Elements(numeric array=w583) -> (sum=w587:sgl)
              n120 = Divide(x=w587, y=1.0) -> (x/y=→"DER8 AC Line-Line Voltage":dbl)
              n121 = Divide(x=w584, y=sgl 1000.0) -> (x/y=→"DER8 Real Power":sgl)
              "DER8 State" <- w591
              "DER8 DC Voltage" <- w590
              "DER8 Logged" <- w592
              "DER8 State of Charge" <- w589
              "DER8 State of Charge Figure" <- w589
            }
            frame 9 {
              n122 = Add Array Elements(numeric array=w596) -> (sum=w598:sgl)
              n123 = Divide(x=w598, y=1.0) -> (x/y=→"DER9 AC Line-Line Votlage":dbl)
              n124 = Divide(x=w594, y=sgl 1000.0) -> (x/y=→"DER9 Real Power":sgl)
              "DER9 State" <- w602
              "DER9 logged" <- w603
              "DER9 Across Variable" <- w601
              "DER9 State of Charge Figure" <- w600
              "DER9 State of Charge" <- w600
            }
            frame 10 {
              n125 = Add Array Elements(numeric array=w606) -> (sum=w609:sgl)
              n126 = Divide(x=w609, y=1.0) -> (x/y=→"DER10 AC Line-Line Voltage":dbl)
              n127 = Divide(x=w607, y=sgl 1000.0) -> (x/y=→"DER10 Real Power":sgl)
              "DER10 State" <- w612
              "DER10 DC Voltage" <- w614
              "DER10 Logged" <- w613
              "DER10 State of Charge Figure" <- w611
              "DER10 State of Charge" <- w611
            }
            frame 11 {
              "DER11 logged" <- w617
              "DER11 State" <- w616
              "DER11 Across Variable" <- w615
              "DER11 State of Charge" <- w618
              "DER11 State of Charge Figure" <- w618
            }
            frame 12 {
              "DER12 State" <- w621
              "DER12 Logged" <- w620
              "DER12 DC Voltage" <- w622
              "DER12 State of Charge" <- w619
              "DER12State of Charge Figure" <- w619
            }
          }
        }
        n128 = local write "SYS Status"("Processing" ("Status")) -> ()
        n129 = Wait Until Next ms Multiple(millisecond multiple=u32 250) -> ()  [unwired: 1 out]
      }
      frame 2 {
        n130 = local read "SYS Current Time"() -> (w624:dbl)
        n131 = local write "SYS Status"("Saving" ("Status")) -> ()
        n132 = Build Array(w624) -> (w628:dbl[])
        n133 = Reshape Array(w628, 19 ("dimension size")) -> (w627:dbl[])
        n134 = Array To Spreadsheet String(array=w627, 3:"%f" ("format string")) -> (spreadsheet string=w633:string)  [unwired: 1 in]
        n135 = Write to Text File(file (use dialog)=w630, text=w633, error in=w629) -> (refnum out=w632:refnum<file>, error out=w631:errorcluster)  [unwired: 1 in, 1 out]
        n136 = Wait Until Next ms Multiple(millisecond multiple=u32 250) -> ()  [unwired: 1 out]
      }
      frame 11 {
        n137 = local read "SYS DER Index"() -> (w638:i32)
        n138 = Index Array(array=w642, index=w638) -> (element=w647:T5)
        n139 = Unbundle(w647) -> ("Modbus master out"=w646:refnum<class "Modbus Master.lvclass">, "error out"=w645:errorcluster)
        n140 = local write "SYS Status"("Start" ("Status")) -> ()
        n141 = call-dynamic "Write Single Holding Register.vi"("error in (no error)"=w645, "holding register value"=u16 1, "address"=u16 2032 ("starting address"), "Modbus master in"=w646) -> ("error out"=w643:errorcluster, "Modbus master out"=w644:refnum<class "Modbus Master.lvclass">)  [unwired: 6 in]
        n142 = Bundle("Modbus master out"=w644, "error out"=w643) -> (w641:T5)  [unwired: 1 in]
        n143 = Wait Until Next ms Multiple(millisecond multiple=u32 250) -> ()  [unwired: 1 out]
        n144 = Replace Array Subset(array=w642, new element=w641, index=w638) -> (w640:T3)
      }
      frame 12 {
        n145 = local read "SYS DER Index"() -> (w653:i32)
        n146 = Index Array(array=w655, index=w653) -> (element=w661:T5)
        n147 = Unbundle(w661) -> ("Modbus master out"=w660:refnum<class "Modbus Master.lvclass">, "error out"=w659:errorcluster)
        n148 = local write "SYS Status"("Stop" ("Status")) -> ()
        n149 = call-dynamic "Write Single Holding Register.vi"("error in (no error)"=w659, "holding register value"=u16 0, "address"=u16 2032 ("starting address"), "Modbus master in"=w660) -> ("error out"=w657:errorcluster, "Modbus master out"=w658:refnum<class "Modbus Master.lvclass">)  [unwired: 6 in]
        n150 = Bundle("Modbus master out"=w658, "error out"=w657) -> (w656:T5)  [unwired: 1 in]
        n151 = Replace Array Subset(array=w655, new element=w656, index=w653) -> (w654:T3)
        n152 = Wait Until Next ms Multiple(millisecond multiple=u32 250) -> ()  [unwired: 1 out]
      }
      frame 13 {
        n153 = local read "SYS DER Index"() -> (w666:i32)
        n154 = String To Byte Array(string="HEILA") -> (unsigned byte array=w681:u8[])
        n155 = Index Array(array=w675, index=w666) -> (element=w677:T5)
        n156 = for {
          N: 16 -> [_]
          tunnel: w681 -> [w692]
          tunnel: [w691] -> w669 mode=indexing
          i -> [w687]
          n157 = Multiply(x=w687, y=2) -> (x*y=w688:i32)
          n158 = Increment(x=w688) -> (x+1=w689:i32)
          n159 = Index Array(array=w692, index #1=w688, index #2=w689) -> (element #1=w686:u8, element #2=w684:u8)
          n160 = To Unsigned Byte Integer(number=w686) -> (unsigned 8bit integer=w685:u8)
          n161 = To Unsigned Byte Integer(number=w684) -> (unsigned 8bit integer=w683:u8)
          n162 = Join Numbers(hi=w685, lo=w683) -> ((hi.lo)=w691:u16)
        }
        n163 = Unbundle(w677) -> ("Modbus master out"=w670:refnum<class "Modbus Master.lvclass">, "error out"=w676:errorcluster)
        n164 = call-dynamic "Write Multiple Holding Registers.vi"("error in (no error)"=w676, "holding register values"=w669, "starting address"=u16 2000, "Modbus master in"=w670) -> ("error out"=w673:errorcluster, "Modbus master out"=w674:refnum<class "Modbus Master.lvclass">)  [unwired: 6 in]
        n165 = local write "SYS Status"("Login" ("Status")) -> ()
        n166 = Bundle("Modbus master out"=w674, "error out"=w673) -> (w672:T5)  [unwired: 1 in]
        n167 = Replace Array Subset(array=w675, new element=w672, index=w666) -> (w671:T3)
        n168 = Wait Until Next ms Multiple(millisecond multiple=u32 250) -> ()  [unwired: 1 out]
      }
      frame 14 {
        n169 = local read "SYS DER Index"() -> (w696:i32)
        n170 = Index Array(array=w705, index=w696) -> (element=w706:T5)
        n171 = local read "data"() -> (w693:T1)
        n172 = Unbundle By Name(w693) -> ("Variable 1 Setpoint"=w694:sgl)
        n173 = Type Cast(type=u32 0, x=w694) -> (*(type *) &x=w711:u32)
        n174 = Split Number(x=w711) -> (hi(x)=w709:u16, lo(x)=w708:u16)
        n175 = Unbundle(w706) -> ("Modbus master out"=w703:refnum<class "Modbus Master.lvclass">, "error out"=w702:errorcluster)
        n176 = Build Array(w709, w708) -> (w697:u16[])
        n177 = call-dynamic "Write Multiple Holding Registers.vi"("error in (no error)"=w702, "holding register values"=w697, "starting address"=u16 2036, "Modbus master in"=w703) -> ("error out"=w700:errorcluster, "Modbus master out"=w701:refnum<class "Modbus Master.lvclass">)  [unwired: 6 in]
        n178 = local write "SYS Status"("Set Real Power" ("Status")) -> ()
        n179 = Bundle("Modbus master out"=w701, "error out"=w700) -> (w699:T5)  [unwired: 1 in]
        n180 = Replace Array Subset(array=w705, new element=w699, index=w696) -> (w704:T3)
        n181 = Wait Until Next ms Multiple(millisecond multiple=u32 10) -> ()  [unwired: 1 out]
      }
      frame 15 {
        n182 = local read "SYS DER Index"() -> (w715:i32)
        n183 = local read "data"() -> (w714:T1)
        n184 = Index Array(array=w716, index=w715) -> (element=w725:T5)
        n185 = Unbundle By Name(w714) -> ("Variable 2 Setpoint"=w713:sgl)
        n186 = Type Cast(type=u32 0, x=w713) -> (*(type *) &x=w729:u32)
        n187 = Split Number(x=w729) -> (hi(x)=w727:u16, lo(x)=w726:u16)
        n188 = Unbundle(w725) -> ("Modbus master out"=w724:refnum<class "Modbus Master.lvclass">, "error out"=w723:errorcluster)
        n189 = Build Array(w727, w726) -> (w718:u16[])
        n190 = call-dynamic "Write Multiple Holding Registers.vi"("error in (no error)"=w723, "holding register values"=w718, "starting address"=u16 2038, "Modbus master in"=w724) -> ("error out"=w721:errorcluster, "Modbus master out"=w722:refnum<class "Modbus Master.lvclass">)  [unwired: 6 in]
        n191 = Bundle("Modbus master out"=w722, "error out"=w721) -> (w720:T5)  [unwired: 1 in]
        n192 = Replace Array Subset(array=w716, new element=w720, index=w715) -> (w717:T3)
        n193 = Wait Until Next ms Multiple(millisecond multiple=u32 50) -> ()  [unwired: 1 out]
      }
      frame 16 {
        # "V"
        n194 = local read "SYS DER Index"() -> (w734:i32)
        n195 = local read "data"() -> (w733:T1)
        n196 = Index Array(array=w736, index=w734) -> (element=w744:T5)
        n197 = Unbundle By Name(w733) -> ("Variable 1 Setpoint"=w732:sgl)
        n198 = Type Cast(type=u32 0, x=w732) -> (*(type *) &x=w748:u32)
        n199 = Split Number(x=w748) -> (hi(x)=w746:u16, lo(x)=w745:u16)
        n200 = Unbundle(w744) -> ("Modbus master out"=w743:refnum<class "Modbus Master.lvclass">, "error out"=w742:errorcluster)
        n201 = Build Array(w746, w745) -> (w737:u16[])
        n202 = call-dynamic "Write Multiple Holding Registers.vi"("error in (no error)"=w742, "holding register values"=w737, "starting address"=u16 2040, "Modbus master in"=w743) -> ("error out"=w740:errorcluster, "Modbus master out"=w741:refnum<class "Modbus Master.lvclass">)  [unwired: 6 in]
        n203 = Bundle("Modbus master out"=w741, "error out"=w740) -> (w739:T5)  [unwired: 1 in]
        n204 = Replace Array Subset(array=w736, new element=w739, index=w734) -> (w735:T3)
        n205 = Wait Until Next ms Multiple(millisecond multiple=u32 50) -> ()  [unwired: 1 out]
      }
      frame 17 {
        n206 = local read "SYS DER Index"() -> (w753:i32)
        n207 = local read "data"() -> (w752:T1)
        n208 = Index Array(array=w755, index=w753) -> (element=w763:T5)
        n209 = Unbundle By Name(w752) -> ("Variable 2 Setpoint"=w751:sgl)
        n210 = Type Cast(type=u32 0, x=w751) -> (*(type *) &x=w767:u32)
        n211 = Split Number(x=w767) -> (hi(x)=w765:u16, lo(x)=w764:u16)
        n212 = Unbundle(w763) -> ("Modbus master out"=w762:refnum<class "Modbus Master.lvclass">, "error out"=w761:errorcluster)
        n213 = Build Array(w765, w764) -> (w756:u16[])
        n214 = call-dynamic "Write Multiple Holding Registers.vi"("error in (no error)"=w761, "holding register values"=w756, "starting address"=u16 2042, "Modbus master in"=w762) -> ("error out"=w759:errorcluster, "Modbus master out"=w760:refnum<class "Modbus Master.lvclass">)  [unwired: 6 in]
        n215 = Bundle("Modbus master out"=w760, "error out"=w759) -> (w758:T5)  [unwired: 1 in]
        n216 = Replace Array Subset(array=w755, new element=w758, index=w753) -> (w754:T3)
        n217 = Wait Until Next ms Multiple(millisecond multiple=u32 250) -> ()  [unwired: 1 out]
      }
      frame 1000 {
        n218 = property class="VI"(reference=w771) -> ("Exec.State"=w772:T6)  [unwired: 1 in, 2 out]
        n219 = case shown="\"Idle\"" w772 {
          tunnel: w773 -> [_ w787 _ _]
          tunnel: w771 -> [_ w777 w796 w798]
          tunnel: [0 0 1000 1000] -> w770
          frame "Bad", Default {
          }
          frame "Idle" {
            n220 = invoke class="VI" method="Run VI"(reference=w777, "Wait until done"=FALSE ("Wait Until Done"), "Auto Dispose Ref"=FALSE ("Auto Dispose Reference")) -> (reference out=w783:refnum<vi>)  [unwired: 2 in, 4 out]
            n221 = local read "SYS DER Index"() -> (w790:i32)
            n222 = invoke class="VI" method="FP.Open"(reference=w783, "Activate"=TRUE ("Activate?"), "State"=T4."Standard") -> (reference out=w782:refnum<vi>)  [unwired: 2 in, 4 out]
            n223 = To Variant(anything=w790) -> (Variant=w792:variant)
            n224 = invoke class="VI" method="Ctrl Val.Set"(reference=w782, "Control Name"="DER", "Value"=w792) -> (reference out=w788:refnum<vi>)  [unwired: 2 in, 4 out]
            n225 = To Variant(anything=w787) -> (Variant=w789:variant)
            n226 = invoke class="VI" method="Ctrl Val.Set"(reference=w788, "Control Name"="Event", "Value"=w789) -> (reference out=w779:refnum<vi>)  [unwired: 2 in, 4 out]
            n227 = To Variant(anything="DER List") -> (Variant=w781:variant)
            n228 = invoke class="VI" method="Ctrl Val.Set"(reference=w779, "Control Name"="DER Names", "Value"=w781) -> ()  [unwired: 2 in, 5 out]
          }
          frame "Run top level" {
            n229 = invoke class="VI" method="Abort VI"(reference=w796) -> ()  [unwired: 2 in, 3 out]
          }
          frame "Running" {
            n230 = invoke class="VI" method="Abort VI"(reference=w798) -> ()  [unwired: 2 in, 3 out]
          }
        }
      }
      frame 1001 {
        n231 = property class="VI"(reference=w799) -> ("Exec.State"=w801:T6)  [unwired: 1 in, 2 out]
        n232 = case shown="\"Idle\"" w801 {
          tunnel: w799 -> [_ w810 w820 w822]
          tunnel: [0 0 1000 1000] -> w800
          frame "Bad", Default {
          }
          frame "Idle" {
            n233 = invoke class="VI" method="Run VI"(reference=w810, "Wait until done"=FALSE ("Wait Until Done"), "Auto Dispose Ref"=FALSE ("Auto Dispose Reference")) -> (reference out=w806:refnum<vi>)  [unwired: 2 in, 4 out]
            n234 = local read "SYS DER Index"() -> (w816:i32)
            n235 = invoke class="VI" method="FP.Open"(reference=w806, "Activate"=TRUE ("Activate?"), "State"=T4."Standard") -> (reference out=w807:refnum<vi>)  [unwired: 2 in, 4 out]
            n236 = To Variant(anything=w816) -> (Variant=w818:variant)
            n237 = invoke class="VI" method="Ctrl Val.Set"(reference=w807, "Control Name"="DER", "Value"=w818) -> (reference out=w811:refnum<vi>)  [unwired: 2 in, 4 out]
            n238 = local read "DER List"() -> (w812:string[])
            n239 = To Variant(anything=w812) -> (Variant=w814:variant)
            n240 = invoke class="VI" method="Ctrl Val.Set"(reference=w811, "Control Name"="DER Names", "Value"=w814) -> ()  [unwired: 2 in, 5 out]
          }
          frame "Run top level" {
            n241 = invoke class="VI" method="Abort VI"(reference=w820) -> ()  [unwired: 2 in, 3 out]
          }
          frame "Running" {
            n242 = invoke class="VI" method="Abort VI"(reference=w822) -> ()  [unwired: 2 in, 3 out]
          }
        }
      }
    }
    n243 = local read "ALL Real Power"() -> (w107:sgl[])
    n244 = for {
      tunnel: w107 -> [w123] mode=indexing
      i -> [w128]
      n245 = Greater?(x=w123, y=sgl 200.0) -> (0:w136:bool)
      n246 = Less?(x=w123, y=sgl -200.0) -> (x < y?=w135:bool)
      n247 = Greater?(x=w123, y=sgl 1000.0) -> (0:w122:bool)
      n248 = Less?(x=w123, y=sgl -1000.0) -> (x < y?=w121:bool)
      n249 = Greater?(x=w123, y=sgl 5000.0) -> (0:w120:bool)
      n250 = Less?(x=w123, y=sgl -5000.0) -> (x < y?=w119:bool)
      n251 = Build Array(w136, w135, w122, w121, w120, w119) -> (w134:bool[])
      n252 = local read "SYS Iteration"() -> (w130:i32)
      n253 = Boolean Array To Number(Boolean array=w134) -> (number=w132:u32)
      n254 = Quotient & Remainder(x=w130, y=3) -> (x-y*floor(x/y)=w129:i32)  [unwired: 1 out]
      n255 = case shown="42" w132 {
        tunnel: [0 ("x") w143 w169 w196 w223 w251 w279] -> w133
        tunnel: w129 -> [_ w141 w168 w194 w221 w249 w277]
        tunnel: w128 -> [_ w140 w166 w197 w225 w253 w281]
        frame 0, Default {
        }
        frame 1 {
          # "> 500W"
          n256 = case shown="4" w140 {
            tunnel: [1 ("x") 1 ("x") 4 ("x") 1 ("x") 1 ("x") 4 ("x") 1 ("x") 4 ("x") 1 ("x") 4 ("x") 1 ("x") 4 ("x") 1 ("x") 4 ("x") 1 ("x") 1 ("x") 4 ("x") 4 ("x") 1 ("x") 1 ("x") 1 ("x") 1 ("x")] -> w142
            frame 0, Default {
            }
            frame 1 {
            }
            frame 2 {
            }
            frame 3 {
            }
            frame 4 {
            }
            frame 5 {
            }
            frame 6 {
            }
            frame 7 {
            }
            frame 8 {
            }
            frame 9 {
            }
            frame 10 {
            }
            frame 11 {
            }
            frame 12 {
            }
            frame 13 {
            }
            frame 14 {
            }
            frame 15 {
            }
            frame 16 {
            }
            frame 17 {
            }
            frame 18 {
            }
            frame 19 {
            }
            frame 20 {
            }
            frame 21 {
            }
          }
          n257 = Add(x=w142, y=w141) -> (x+y=w143:i32)
        }
        frame 2 {
          # "< -500W"
          n258 = case shown="4" w166 {
            tunnel: [4 ("x") 4 ("x") 1 ("x") 4 ("x") 4 ("x") 1 ("x") 4 ("x") 1 ("x") 4 ("x") 1 ("x") 4 ("x") 1 ("x") 4 ("x") 1 ("x") 4 ("x") 4 ("x") 1 ("x") 1 ("x") 4 ("x") 4 ("x") 4 ("x") 4 ("x")] -> w167
            frame 0, Default {
            }
            frame 1 {
            }
            frame 2 {
            }
            frame 3 {
            }
            frame 4 {
            }
            frame 5 {
            }
            frame 6 {
            }
            frame 7 {
            }
            frame 8 {
            }
            frame 9 {
            }
            frame 10 {
            }
            frame 11 {
            }
            frame 12 {
            }
            frame 13 {
            }
            frame 14 {
            }
            frame 15 {
            }
            frame 16 {
            }
            frame 17 {
            }
            frame 18 {
            }
            frame 19 {
            }
            frame 20 {
            }
            frame 21 {
            }
          }
          n259 = Add(x=w167, y=w168) -> (x+y=w169:i32)
        }
        frame 5 {
          # "> 2000W"
          n260 = case shown="4" w197 {
            tunnel: [1 ("x") 1 ("x") 4 ("x") 1 ("x") 1 ("x") 4 ("x") 1 ("x") 4 ("x") 1 ("x") 4 ("x") 1 ("x") 4 ("x") 1 ("x") 4 ("x") 1 ("x") 1 ("x") 4 ("x") 4 ("x") 1 ("x") 1 ("x") 1 ("x") 1 ("x")] -> w195
            frame 0, Default {
            }
            frame 1 {
            }
            frame 2 {
            }
            frame 3 {
            }
            frame 4 {
            }
            frame 5 {
            }
            frame 6 {
            }
            frame 7 {
            }
            frame 8 {
            }
            frame 9 {
            }
            frame 10 {
            }
            frame 11 {
            }
            frame 12 {
            }
            frame 13 {
            }
            frame 14 {
            }
            frame 15 {
            }
            frame 16 {
            }
            frame 17 {
            }
            frame 18 {
            }
            frame 19 {
            }
            frame 20 {
            }
            frame 21 {
            }
          }
          n261 = Add(x=6, y=w194) -> (x+y=w192:i32)
          n262 = Add(x=w195, y=w192) -> (x+y=w196:i32)
        }
        frame 10 {
          # "< -2000W"
          n263 = case shown="12" w225 {
            tunnel: [4 ("x") 4 ("x") 1 ("x") 4 ("x") 4 ("x") 1 ("x") 4 ("x") 1 ("x") 4 ("x") 1 ("x") 4 ("x") 1 ("x") 4 ("x") 1 ("x") 4 ("x") 4 ("x") 1 ("x") 1 ("x") 4 ("x") 4 ("x") 4 ("x") 4 ("x")] -> w224
            frame 0, Default {
            }
            frame 1 {
            }
            frame 2 {
            }
            frame 3 {
            }
            frame 4 {
            }
            frame 5 {
            }
            frame 6 {
            }
            frame 7 {
            }
            frame 8 {
            }
            frame 9 {
            }
            frame 10 {
            }
            frame 11 {
            }
            frame 12 {
            }
            frame 13 {
            }
            frame 14 {
            }
            frame 15 {
            }
            frame 16 {
            }
            frame 17 {
            }
            frame 18 {
            }
            frame 19 {
            }
            frame 20 {
            }
            frame 21 {
            }
          }
          n264 = Add(x=6, y=w221) -> (x+y=w220:i32)
          n265 = Add(x=w224, y=w220) -> (x+y=w223:i32)
        }
        frame 21 {
          # "> 8000W"
          n266 = case shown="12" w253 {
            tunnel: [1 ("x") 1 ("x") 4 ("x") 1 ("x") 1 ("x") 4 ("x") 1 ("x") 4 ("x") 1 ("x") 4 ("x") 1 ("x") 4 ("x") 1 ("x") 4 ("x") 1 ("x") 1 ("x") 4 ("x") 4 ("x") 1 ("x") 1 ("x") 1 ("x") 1 ("x")] -> w252
            frame 0, Default {
            }
            frame 1 {
            }
            frame 2 {
            }
            frame 3 {
            }
            frame 4 {
            }
            frame 5 {
            }
            frame 6 {
            }
            frame 7 {
            }
            frame 8 {
            }
            frame 9 {
            }
            frame 10 {
            }
            frame 11 {
            }
            frame 12 {
            }
            frame 13 {
            }
            frame 14 {
            }
            frame 15 {
            }
            frame 16 {
            }
            frame 17 {
            }
            frame 18 {
            }
            frame 19 {
            }
            frame 20 {
            }
            frame 21 {
            }
          }
          n267 = Add(x=12, y=w249) -> (x+y=w248:i32)
          n268 = Add(x=w252, y=w248) -> (x+y=w251:i32)
        }
        frame 42 {
          # "< -8000W"
          n269 = case shown="12" w281 {
            tunnel: [4 ("x") 4 ("x") 1 ("x") 4 ("x") 4 ("x") 1 ("x") 4 ("x") 1 ("x") 4 ("x") 1 ("x") 4 ("x") 1 ("x") 4 ("x") 1 ("x") 4 ("x") 4 ("x") 1 ("x") 1 ("x") 4 ("x") 4 ("x") 4 ("x") 4 ("x")] -> w280
            frame 0, Default {
            }
            frame 1 {
            }
            frame 2 {
            }
            frame 3 {
            }
            frame 4 {
            }
            frame 5 {
            }
            frame 6 {
            }
            frame 7 {
            }
            frame 8 {
            }
            frame 9 {
            }
            frame 10 {
            }
            frame 11 {
            }
            frame 12 {
            }
            frame 13 {
            }
            frame 14 {
            }
            frame 15 {
            }
            frame 16 {
            }
            frame 17 {
            }
            frame 18 {
            }
            frame 19 {
            }
            frame 20 {
            }
            frame 21 {
            }
          }
          n270 = Add(x=12, y=w277) -> (x+y=w276:i32)
          n271 = Add(x=w280, y=w276) -> (x+y=w279:i32)
        }
      }
      n272 = case shown="6" w128 {
        tunnel: w133 -> [w304 w305 w306 w307 w308 w309 w310 w311 w312 w313 w314 w315 w316]
        frame 0, Default {
          "DER0 Flow" <- w304
        }
        frame 1 {
          "DER1 Flow" <- w305
        }
        frame 2 {
          "DER2 Flow" <- w306
        }
        frame 3 {
          "DER3 Flow" <- w307
        }
        frame 4 {
          "DER4 Flow" <- w308
        }
        frame 5 {
          "DER5 Flow" <- w309
        }
        frame 6 {
          "DER6 Flow" <- w310
        }
        frame 7 {
          "DER7 Flow" <- w311
        }
        frame 8 {
          "DER8 Flow" <- w312
        }
        frame 9 {
          "DER9 Flow" <- w313
        }
        frame 10 {
          "DER10 Flow" <- w314
        }
        frame 11 {
          "DER11 Flow" <- w315
        }
        frame 12 {
          "DER12 Flow" <- w316
        }
      }
    }
    n273 = local write "SYS Case"(w82) -> ()
    n274 = for {
      tunnel: w111 -> [w319] mode=indexing
      tunnel: [w318] -> w110 mode=indexing
      tunnel: [w319] -> w108 mode=indexing
      tunnel: [w317] -> w109 mode=indexing
      n275 = Unbundle(w319) -> ("error out"=w318:errorcluster)  [unwired: 1 out]
      n276 = Unbundle By Name(w318) -> ("status"=w317:bool)
    }
    "ALL DER Current Error" <- w110
    "ALL Error Indicator" <- w109
  }
  n277 = Close File(refnum=w22, error in=w21) -> (error out=→"error out 3":errorcluster)  [unwired: 1 out]
  n278 = for {
    tunnel: w27 -> [w826] mode=indexing
    tunnel: [w823] -> w31 mode=indexing
    n279 = Unbundle(w826) -> ("Modbus master out"=w825:refnum<class "Modbus Master.lvclass">, "error out"=w824:errorcluster)
    n280 = call-dynamic "Close.vi"("error in (no error)"=w824, "Modbus master in"=w825) -> ("error out"=w823:errorcluster)  [unwired: 9 in]
  }
  "ALL DER Final Error" <- w31
  n281 = Unregister For Events(event registration refnum=w9) -> ()  [unwired: 1 in, 1 out]
  n282 = Destroy User Event(user event=w8) -> ()  [unwired: 1 in, 1 out]
  n283 = Destroy User Event(user event=w5) -> ()  [unwired: 1 in, 1 out]
  "SYS Iteration" <- 0
  "SYS DER Index" <- 0 ("DER Index")
  "SYS Status" <- "Initializing" ("Sys Status")
  "SYS Case" <- 0 ("SYS Case")
